vi "offset_multiplier.vi"(1 "axis info":T2={"samples"=128, "end"=1.0, "start"=0.0}) -> (0 "offset & multiplier":T1)   [LabVIEW 2019, in "Mandelbrot.lvlib"]
uses:
  Mandelbrot.lvlib
  axis_info.ctl
  <vilib>/Utility/miscctls.llb/LVOffsetAndMultiplierTypeDef.ctl
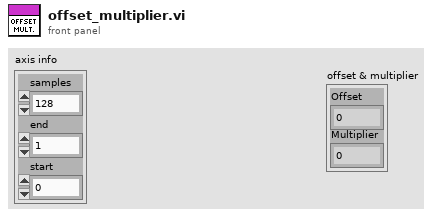
[diagram p1: front panel]
types:
  T1 = typedef "LVOffsetAndMultiplierTypeDef.ctl" = cluster{"Offset":dbl, "Multiplier":dbl}
  T2 = typedef "Mandelbrot.lvlib/axis_info.ctl" = cluster{"samples":i32, "end":dbl, "start":dbl}
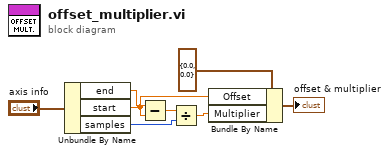
[diagram p0: block diagram]
diagram:
  n1 = Unbundle By Name("axis info") -> ("end"=w7:dbl, "start"=w3:dbl, "samples"=w5:i32)
  n2 = Subtract(x=w7, y=w3) -> (x-y=w6:dbl)
  n3 = Divide(x=w6, y=w5) -> (x/y=w2:dbl)
  n4 = Bundle By Name(cluster=T1 {"Offset"=0.0, "Multiplier"=0.0} ("X Scale.Offset and Multiplier"), "Offset"=w3, "Multiplier"=w2) -> (→"offset & multiplier":T1)
